vi "Generate ROI overlay.vi"(10 "POI on selected plane":dbl[][](array[numeric]), 11 "Refnum in":T1) -> (3 "Refnum out":T1)   [LabVIEW 2020]
uses:
  <vilib>/vision/Image Controls.llb/IMAQ Image.ctl
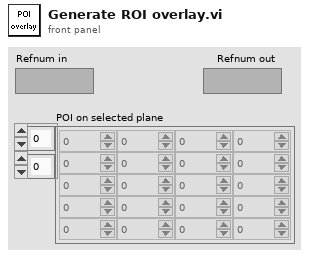
[diagram p1: front panel]
types:
  T1 = typedef "IMAQ Image.ctl" = refnum<image>
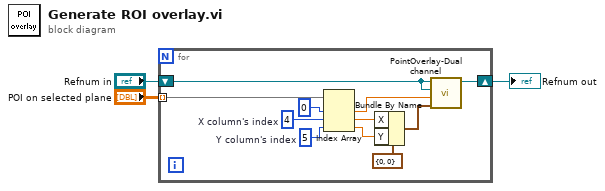
[diagram p0: block diagram]
diagram:
  n1 = for {
    shift-right: [w14] -> w3
    shift-left: "Refnum in" -> [w7]
    tunnel: "POI on selected plane" -> [w13] mode=indexing
    w4 = 5  # Y column's index
    w5 = 4  # X column's index
    n2 = Index Array(array=w13, index #1=0 ("index"), index #2=w5, index #3=w4) -> (element #1=w10:dbl, element #2=w9:dbl, element #3=w8:dbl)
    n3 = Bundle By Name(cluster=cluster{"X":i32, "Y":i32} {"X"=0, "Y"=0} ("Coordinates"), "X"=w9, "Y"=w8) -> (w11:cluster{"X":i32, "Y":i32})
    n4 = call "PointOverlay-Dual channel.vi"("Coordinates"=w11, "Count"=w10, "Image2"=w7, "Image1"=w7) -> ("Image1 Out"=w14:T1)  [unwired: 6 in, 1 out]
  }
  "Refnum out" <- w3
